vi "ArgumentManipulation.vi"(11 "String":string) -> (3 "Argument":string, 5 "Property or SSM":string)   [LabVIEW 2018]
doc: "This VI manipulates the information coming from the command string."
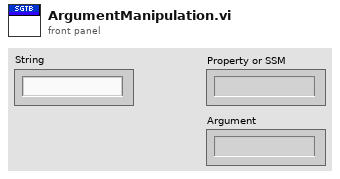
[diagram p1: front panel]
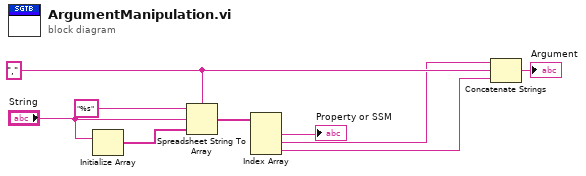
[diagram p0: block diagram]
diagram:
  w5 = "," ("delimiter (Tab)")
  n1 = Initialize Array("String") -> (w9:string[])  [unwired: 1 in]
  n2 = Spreadsheet String To Array(delimiter (Tab)=w5, format string="%s", spreadsheet string="String", array type (2D Dbl)=w9) -> (array=w7:string[])
  n3 = Index Array(array=w7) -> (element #1=→"Property or SSM":string, element #2=w4:string, element #3=w3:string)  [unwired: 3 in]
  n4 = Concatenate Strings(w4, w5, w3) -> (→"Argument":string)
